vi "CollectISEOnly.vi"() -> ()   [LabVIEW 2016]
uses:
  <vilib>/Utility/file.llb/Write Delimited Spreadsheet (string).vi
  <vilib>/Utility/file.llb/Write Delimited Spreadsheet (DBL).vi
panel:
  out "Waveform Chart":T1(graph)
  out "Equilibrium?":bool[][](array[boolean])=[[FALSE, TRUE, FALSE, FALSE, TRUE, TRUE]]
  in  "Stabilzation \nCriterion (mV/min)":dbl=0.4
  in  "Differential Window Size (sec)":i64=5
  in  "Array":string[][](array[string])=[["M6AI2", "M6AI4", "M6AI6", "M6AI16", "M6AI18", "M6AI20", "Calculated", "Calculated", "Calculated"], ["NH4+", "Ca2+", "K+", "Na+", "Cl-", "NO3-", "[K+]", "[Na+]", "[NH4+]"]]
  in  "error in":errorcluster
  out "error out":errorcluster={"status"=TRUE, "code"=7, "source"="Open/Create/Replace File in Write Spreadsheet String.vi->Write Delimited Spreadsheet (string).vi->CollectISEOnly.vi<APPEND>\n/u/ISE_Measurements_06042018_235154.csv"}
  in  "File Name:":string="ISE_Measurements"
  out "new file path (Not A Path if cancelled)":path
  in  "stop":bool
  out "All data":dbl[][](array[numeric])=[[1528127514.1565871, 0.0, 0.0, 0.0, 0.0, 0.0, 0.0, inf, nan, nan], [1528127515.158382, 0.0, 0.0, 0.0, 0.0, 0.0, 0.0, inf, nan, nan], [1528127516.159772, 0.0, 0.0, 0.0, 0.0, 0.0, 0.0, inf, nan, nan], [1528127517.1598802, 0.0, 0.0, 0.0, 0.0, 0.0, 0.0, inf, nan, nan], [1528127518.1617708, 0.0, 0.0, 0.0, 0.0, 0.0, 0.0, inf, nan, nan]] format="%#3.4f"
  out "Saving?":bool=TRUE
  out "File Headers":string[][](array[string])=[["Unix Time Code - 8hrs", "M6AI2", "M6AI4", "M6AI6", "M6AI16", "M6AI18", "M6AI20"], ["Unix Time Code - 8hrs", "NH4+", "Ca2+", "K+", "Na+", "Cl-", "NO3-"]]
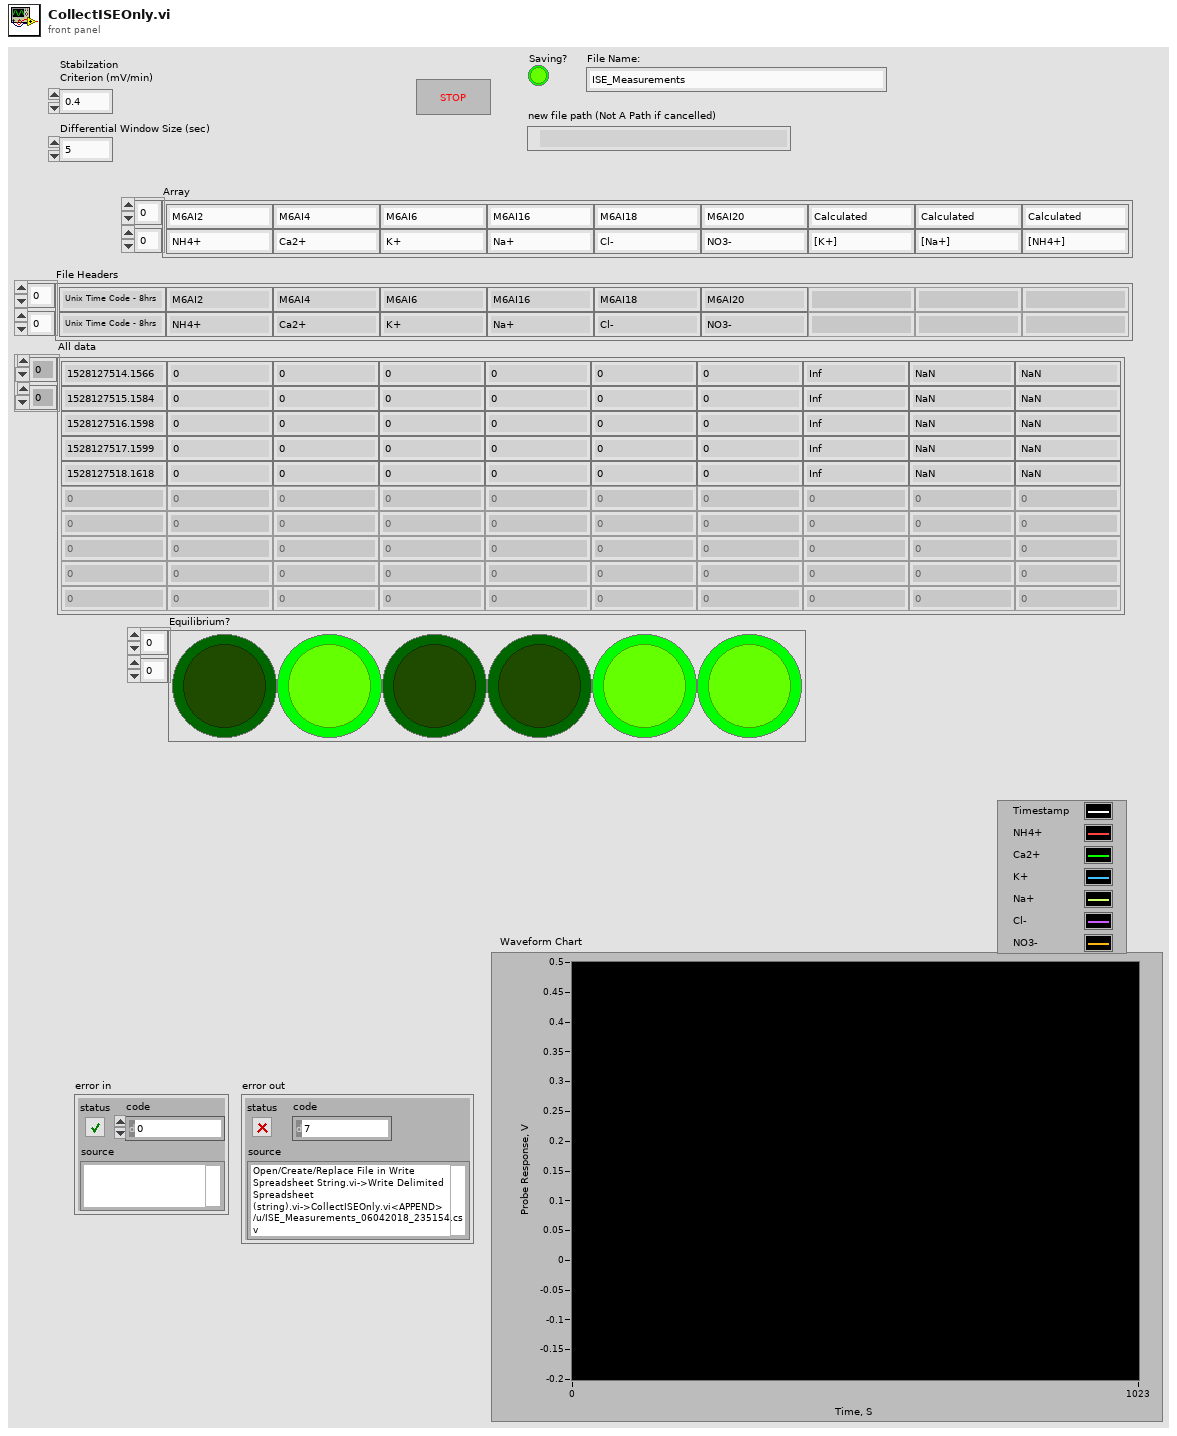
[diagram p1: front panel]
types:
  T1 = cluster{"[0]":dbl, "[1]":dbl, "[2]":dbl, "[3]":dbl, "[4]":dbl, "[5]":dbl, "[6]":dbl, "[7]":dbl, "[8]":dbl}
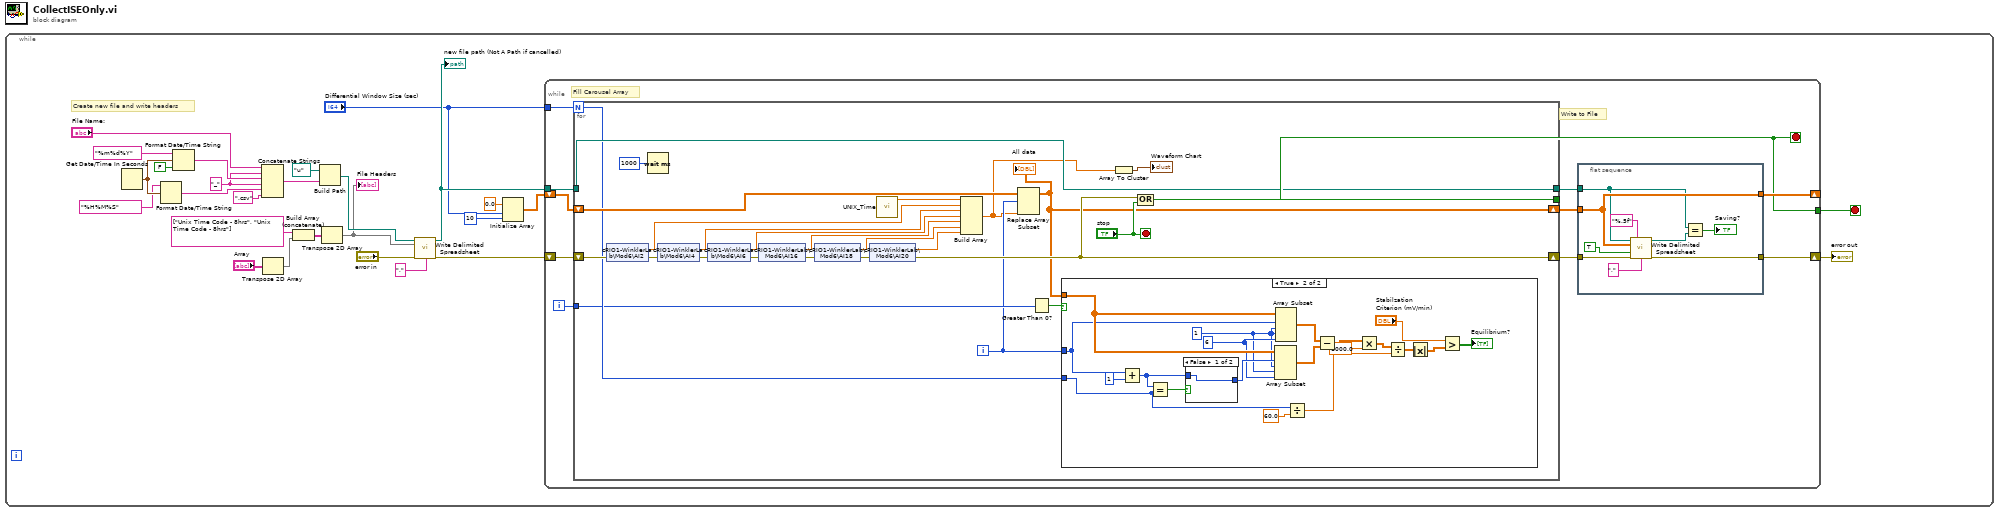
[diagram p0: block diagram]
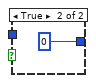
[diagram p3: hidden frame]
diagram:
  n1 = while {
    stop <- w2 stop-if-true
    w16 = "_" ("string")
    # "Create new file and write headers"
    n2 = Get Date/Time In Seconds() -> (seconds since 1Jan1904=w21:timestamp)
    n3 = Format Date/Time String(time format string (%c)="%H%M%S", seconds (now)=w21) -> (date/time string=w15:string)  [unwired: 1 in]
    n4 = Format Date/Time String(time format string (%c)="%m%d%Y", seconds (now)=w21, UTC format=FALSE) -> (date/time string=w17:string)
    n5 = Concatenate Strings("File Name:", w16, w17, w16, w15, ".csv" ("string")) -> (w14:string)
    n6 = Transpose 2D Array(2D array="Array") -> (transposed array=w9:string[][])
    n7 = Build Array (concatenate)(string[] ["Unix Time Code - 8hrs", "Unix Time Code - 8hrs"], w9) -> (w10:string[][])
    n8 = Build Path(base path=path "u:/" ("Save to:"), name or relative path=w14) -> (appended path=w23:path)
    n9 = Transpose 2D Array(2D array=w10) -> (transposed array=w8:string[][])
    "File Headers" <- w8
    n10 = call-poly <vilib>:"Write Delimited Spreadsheet.vi"("file path (dialog if empty)"=w23, "2D data"=w8, "error in (no error)"="error in", "delimiter (\\t)"="," ("delimiter (\\t)")) -> ("new file path (Not A Path if cancelled)"=w27:path, "error out"=w26:errorcluster)  [unwired: 10 in]
    "new file path (Not A Path if cancelled)" <- w27
    n11 = Initialize Array(0.0 ("element"), "Differential Window Size (sec)", 10 ("dimension size")) -> (w3:dbl[][])
    n12 = while {
      tunnel: w27 -> [w38]
      shift-right: [w34] -> w11
      shift-left: w26 -> [w37]
      tunnel: "Differential Window Size (sec)" -> [w33]
      shift-right: [w31] -> _
      shift-left: w3 -> [w30]
      tunnel: [w29] -> w2
      i -> [w28]
      stop <- w29 stop-if-true
      # "Fill Carousel Array"
      # "Write to File"
      n13 = for {
        N: w33 -> [w54]
        tunnel: w38 -> [w60]
        tunnel: [w57] -> w29
        shift-right: [w61] -> w35
        shift-left: w37 -> [w72]
        tunnel: [w60] -> w32
        shift-right: [w56] -> w36
        shift-left: w30 -> [w59]
        tunnel: w28 -> [w53]
        i -> [w52]
        stop <- "stop" stop-if-true
        n14 = shared-variable "cRIO1-WinklerLab\\Mod6\\AI2"(error in=w72) -> (w51:dbl, error out=w71:errorcluster)
        n15 = Wait (ms)(milliseconds to wait=u32 1000) -> ()  [unwired: 1 out]
        n16 = shared-variable "cRIO1-WinklerLab\\Mod6\\AI4"(error in=w71) -> (w66:dbl, error out=w70:errorcluster)
        n17 = shared-variable "cRIO1-WinklerLab\\Mod6\\AI6"(error in=w70) -> (w65:dbl, error out=w69:errorcluster)
        n18 = shared-variable "cRIO1-WinklerLab\\Mod6\\AI16"(error in=w69) -> (w64:dbl, error out=w68:errorcluster)
        n19 = shared-variable "cRIO1-WinklerLab\\Mod6\\AI18"(error in=w68) -> (w63:dbl, error out=w67:errorcluster)
        n20 = shared-variable "cRIO1-WinklerLab\\Mod6\\AI20"(error in=w67) -> (w50:dbl, error out=w61:errorcluster)
        n21 = call "UNIX_Time.vi"() -> ("Unix time"=w73:dbl)  [unwired: 10 in, 1 out]
        n22 = Build Array(w73, w51, w66, w65, w64, w63, w50) -> (w49:dbl[])
        n23 = Replace Array Subset(array=w59, new element=w49, index (row)=w52) -> (w56:dbl[][])  [unwired: 1 in]
        "All data" <- w56
        n24 = Greater Than 0?(x=w53) -> (x > 0?=w55:bool)
        n25 = case shown="True" w55 {
          tunnel: w56 -> [_ w93]
          tunnel: w52 -> [_ w92]
          tunnel: w54 -> [_ w82]
          frame False {
          }
          frame True {
            w87 = 6 ("length")
            w81 = 1 ("index")
            n26 = Add(x=w92, y=1) -> (x+y=w88:i32)
            n27 = Equal?(x=w88, y=w82) -> (x = y?=w90:bool)
            n28 = case shown="False" w90 {
              tunnel: [w94 0 ("y")] -> w89
              tunnel: w88 -> [w94 _]
              frame False {
              }
              frame True {
              }
            }
            n29 = Array Subset(array=w93, index (row)=w89, length (row)=w81, index (col)=w81, length (col)=w87) -> (w85:dbl[][])
            n30 = Array Subset(array=w93, index (row)=w92, length (row)=w81, index (col)=w81, length (col)=w87) -> (w86:dbl[][])
            n31 = Divide(x=w82, y=60.0) -> (x/y=w84:dbl)
            n32 = Subtract(x=w86, y=w85) -> (x-y=w77:dbl[][])
            n33 = Multiply(x=w77, y=1000.0) -> (x*y=w78:dbl[][])
            n34 = Divide(x=w78, y=w84) -> (x/y=w74:dbl[][])
            n35 = Absolute Value(x=w74) -> (abs(x)=w75:dbl[][])
            n36 = Greater?(x="Stabilzation \nCriterion (mV/min)", y=w75) -> (0:→"Equilibrium?":bool[][])
          }
        }
        n37 = Array To Cluster(array=w49) -> (cluster=→"Waveform Chart":T1)
        n38 = Compound Arithmetic op=OR(w61, "stop") -> (w57:bool)
      }
      n39 = flat-sequence {
        tunnel: w36 -> [w40]
        tunnel: w35 -> [w47]
        tunnel: [w46] -> w34
        tunnel: w32 -> [w39]
        tunnel: [w40] -> w31
        frame #0 {
          n40 = call-poly <vilib>:"Write Delimited Spreadsheet.vi"("file path (dialog if empty)"=w39, "format (%.3f)"="%.5f", "2D data"=w40, "append to file? (new file:F)"=TRUE, "error in (no error)"=w47, "delimiter (\\t)"="," ("delimiter (\\t)")) -> ("new file path (Not A Path if cancelled)"=w44:path, "error out"=w46:errorcluster)  [unwired: 8 in]
          n41 = Equal?(x=w39, y=w44) -> (x = y?=→"Saving?":bool)
        }
      }
    }
    "error out" <- w11
  }
